vi "SlopeAndValue.vi"(10 "Threshold time":dbl format="%#_13g", 11 "Values History":T1[](array[typedef])) -> (2 "Derivative":dbl, 3 "Value":dbl)   [LabVIEW 2014]
doc: "Returns the the last value of values history and uses a second order interpolating polynomial to estimate the derivative at that last value. Only takes into account points that occur after threshold time"
uses:
  FlappyHeightPoint.ctl
  <vilib>/Analysis/6fits.llb/Curve Fitting Criteria.ctl
  <vilib>/Analysis/polynomials.llb/nth Derivative of Polynomial (DBL).vi
  <vilib>/Analysis/polynomials.llb/Scalar Polynomial Evaluation (DBL).vi
  <vilib>/Analysis/NI_AALPro.lvlib
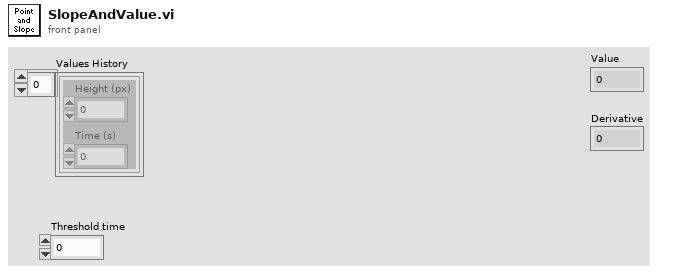
[diagram p1: front panel]
types:
  T1 = typedef "FlappyHeightPoint.ctl" = cluster{"Time (s)":dbl, "Height (px)":dbl}
  T2 = typedef "NI_AALPro.lvlib/Curve Fitting Criteria.ctl" = u16
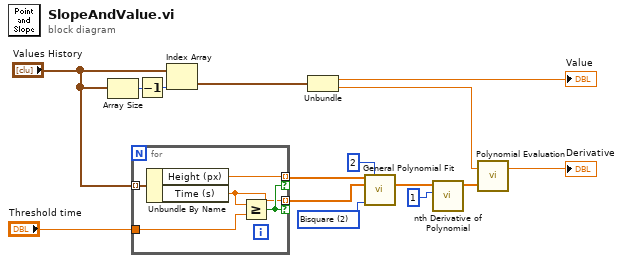
[diagram p0: block diagram]
diagram:
  w6 = T2 2 items=["Least Square", "Least Absolute Residual", "Bisquare"] ("method")
  n1 = Array Size(array="Values History") -> (size(s)=w15:i32)
  n2 = for {
    tunnel: "Values History" -> [w19] mode=indexing
    tunnel: "Threshold time" -> [w20]
    tunnel: [w16] -> w8 mode=indexing if=w17
    tunnel: [w18] -> w9 mode=indexing if=w17
    n3 = Unbundle By Name(w19) -> ("Height (px)"=w18:dbl, "Time (s)"=w16:dbl)
    n4 = Greater Or Equal?(x=w16, y=w20) -> (x >= y?=w17:bool)
  }
  n5 = Decrement(x=w15) -> (x-1=w14:i32)
  n6 = Index Array(array="Values History", index=w14) -> (element=w13:T1)
  n7 = Unbundle(w13) -> ("Time (s)"=→"Value":dbl, "Height (px)"=w2:dbl)
  n8 = call <vilib>:"General Polynomial Fit.vi"("Y"=w9, "polynomial order"=2, "X"=w8, "method"=w6) -> ("Polynomial Coefficients"=w5:dbl[])  [unwired: 8 in, 3 out]
  n9 = call-poly <vilib>:"nth Derivative of Polynomial.vi"("order"=1, "P(x)"=w5) -> ("Nth Derivative of P(x)"=w3:dbl[])  [unwired: 8 in, 1 out]
  n10 = call-poly <vilib>:"Polynomial Evaluation.vi"("P(x)"=w3, "a"=w2) -> ("P(a)"=→"Derivative":dbl)  [unwired: 1 out]
